vi "DashboardGet.vi"(10 "Joystick 2":T1, 11 "Joystick 1":T1) -> ()   [LabVIEW 2018]
uses:
  <vilib>/Rock Robotics/WPI/Joystick/WPI_JoystickDevRef.ctl
  <vilib>/Rock Robotics/WPI/Joystick/WPI_JoystickDeviceEnum.ctl
  RefNumsDriverStation.vi
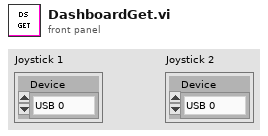
[diagram p1: front panel]
types:
  T1 = typedef "WPI_JoystickDevRef.ctl" = cluster{"Device":T2}
  T2 = typedef "WPI_JoystickDeviceEnum.ctl" = enum16{"USB 0", "USB 1", "USB 2", "USB 3", "USB 4", "USB 5"}
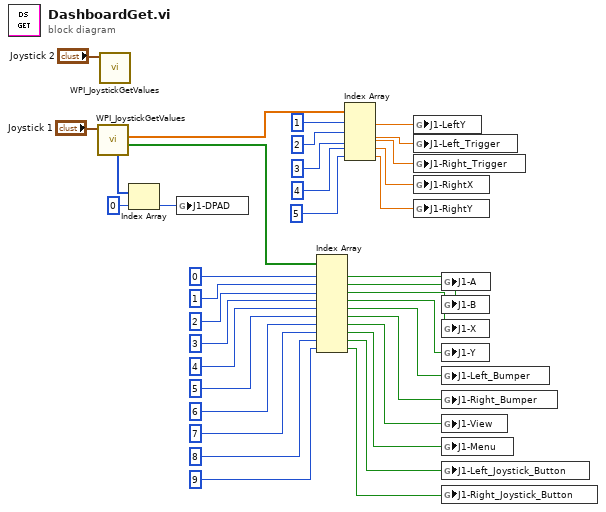
[diagram p0: block diagram]
diagram:
  n1 = call <vilib>:"WPI_JoystickGetValues.vi"("JoystickDevRef"="Joystick 1") -> ("Buttons"=w33:bool[], "Axes"=w34:dbl[], "POVs"=w37:i16[])  [unwired: 6 in, 2 out]
  n2 = call <vilib>:"WPI_JoystickGetValues.vi"("JoystickDevRef"="Joystick 2") -> ()  [unwired: 6 in, 5 out]
  n3 = Index Array(array=w37, index=0) -> (element=w35:i16)
  n4 = global write "RefNumsDriverStation.vi" "J1-DPAD"(w35) -> ()
  n5 = Index Array(array=w33, index #1=0 ("index"), index #2=1 ("index"), index #3=2 ("index"), index #4=3 ("index"), index #5=4 ("index"), index #6=5 ("index"), index #7=6 ("index"), index #8=7 ("index"), index #9=8 ("index"), index #10=9 ("index")) -> (element #1=w24:bool, element #2=w23:bool, element #3=w22:bool, element #4=w21:bool, element #5=w20:bool, element #6=w19:bool, element #7=w18:bool, element #8=w17:bool, element #9=w16:bool, element #10=w4:bool)
  n6 = Index Array(array=w34, index #1=1 ("index"), index #2=2 ("index"), index #3=3 ("index"), index #4=4 ("index"), index #5=5 ("index")) -> (element #1=w32:dbl, element #2=w25:dbl, element #3=w31:dbl, element #4=w30:dbl, element #5=w1:dbl)
  n7 = global write "RefNumsDriverStation.vi" "J1-LeftY"(w32) -> ()
  n8 = global write "RefNumsDriverStation.vi" "J1-Left_Trigger"(w25) -> ()
  n9 = global write "RefNumsDriverStation.vi" "J1-Right_Trigger"(w31) -> ()
  n10 = global write "RefNumsDriverStation.vi" "J1-RightX"(w30) -> ()
  n11 = global write "RefNumsDriverStation.vi" "J1-RightY"(w1) -> ()
  n12 = global write "RefNumsDriverStation.vi" "J1-A"(w24) -> ()
  n13 = global write "RefNumsDriverStation.vi" "J1-B"(w23) -> ()
  n14 = global write "RefNumsDriverStation.vi" "J1-X"(w22) -> ()
  n15 = global write "RefNumsDriverStation.vi" "J1-Y"(w21) -> ()
  n16 = global write "RefNumsDriverStation.vi" "J1-Left_Bumper"(w20) -> ()
  n17 = global write "RefNumsDriverStation.vi" "J1-Right_Bumper"(w19) -> ()
  n18 = global write "RefNumsDriverStation.vi" "J1-View"(w18) -> ()
  n19 = global write "RefNumsDriverStation.vi" "J1-Menu"(w17) -> ()
  n20 = global write "RefNumsDriverStation.vi" "J1-Left_Joystick_Button"(w16) -> ()
  n21 = global write "RefNumsDriverStation.vi" "J1-Right_Joystick_Button"(w4) -> ()
